vi "Max-Min2.vi"(0 "Color Plane (Color Plane Extraction 1)":i32(ring)=3 items=["Red", "Green", "Blue", "Hue", "Saturation", "Luminance", "Value", "Intensity"], 1 "Operator (Lookup Table 1)":T2(ring)=enum."Power X", 2 "X Value (Lookup Table 1)":sgl=2.0, 3 "ROI Descriptors (Quantify 1)":T1(array[cluster])=[{"Global Rectangle"=[0, 0, 160, 120], "Contours"=[{"ID"=enum."External", "Type"=3, "Coordinates"=[0, 0, 160, 120]}]}, {"Global Rectangle"=[18, 13, 28, 23], "Contours"=[{"ID"=enum."External", "Type"=3, "Coordinates"=[18, 13, 28, 23]}]}, {"Global Rectangle"=[77, 13, 87, 23], "Contours"=[{"ID"=enum."External", "Type"=3, "Coordinates"=[77, 13, 87, 23]}]}, {"Global Rectangle"=[135, 12, 145, 23], "Contours"=[{"ID"=enum."External", "Type"=3, "Coordinates"=[135, 12, 145, 23]}]}, {"Global Rectangle"=[18, 53, 28, 64], "Contours"=[{"ID"=enum."External", "Type"=3, "Coordinates"=[18, 53, 28, 64]}]}, {"Global Rectangle"=[77, 53, 87, 64], "Contours"=[{"ID"=enum."External", "Type"=3, "Coordinates"=[77, 53, 87, 64]}]}, {"Global Rectangle"=[137, 54, 146, 64], "Contours"=[{"ID"=enum."External", "Type"=3, "Coordinates"=[137, 54, 146, 64]}]}, {"Global Rectangle"=[18, 92, 28, 102], "Contours"=[{"ID"=enum."External", "Type"=3, "Coordinates"=[18, 92, 28, 102]}]}, {"Global Rectangle"=[77, 90, 87, 100], "Contours"=[{"ID"=enum."External", "Type"=3, "Coordinates"=[77, 90, 87, 100]}]}, {"Global Rectangle"=[136, 88, 146, 99], "Contours"=[{"ID"=enum."External", "Type"=3, "Coordinates"=[136, 88, 146, 99]}]}] {"Contours"."Type" items=["No Selection", "Point", "Line", "Rectangle", "Oval", "Polygon", "Freehand Region", "Annulus", "Unused2", "Unused3", "Broken Line", "Freehand Line", "Rotated Rectangle"]}, 7 "error in":errorcluster) -> (20 "Results (Quantify 1)":sgl[][](array[numeric]) format="%.2f", 27 "error out":errorcluster)   [LabVIEW 2009]
uses:
  <vilib>/vision/NI_Vision_Development_Module.lvlib
panel:
  out "Image Out":T3(plugin-control)
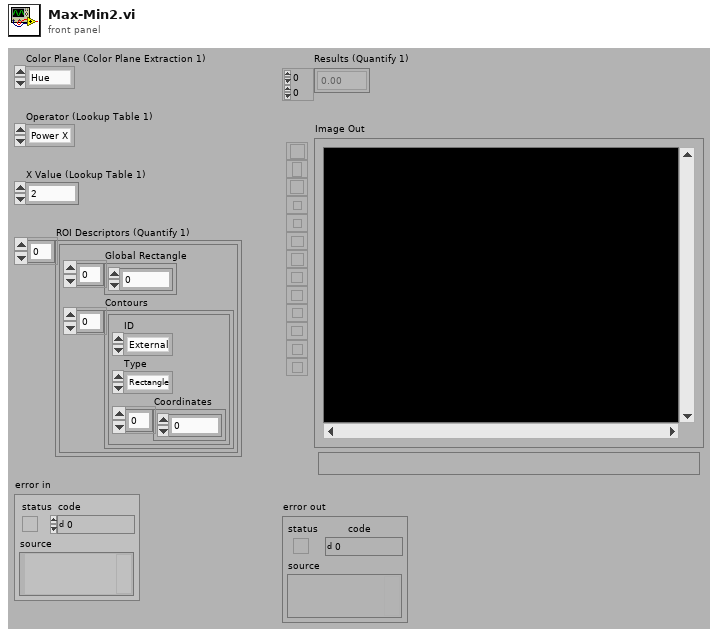
[diagram p1: front panel]
types:
  T1 = cluster{"Global Rectangle":i32[], "Contours":cluster{"ID":enum32{"External", "Internal"}, "Type":u32, "Coordinates":i32[]}[]}[]
  T2 = enum32{"Linear", "Log", "Exp", "Square", "Square root", "Power X", "Power 1/X"}
  T3 = typedef "IMAQ Image.ctl" = refnum<image>
  T4 = typedef "Image Type" = u32
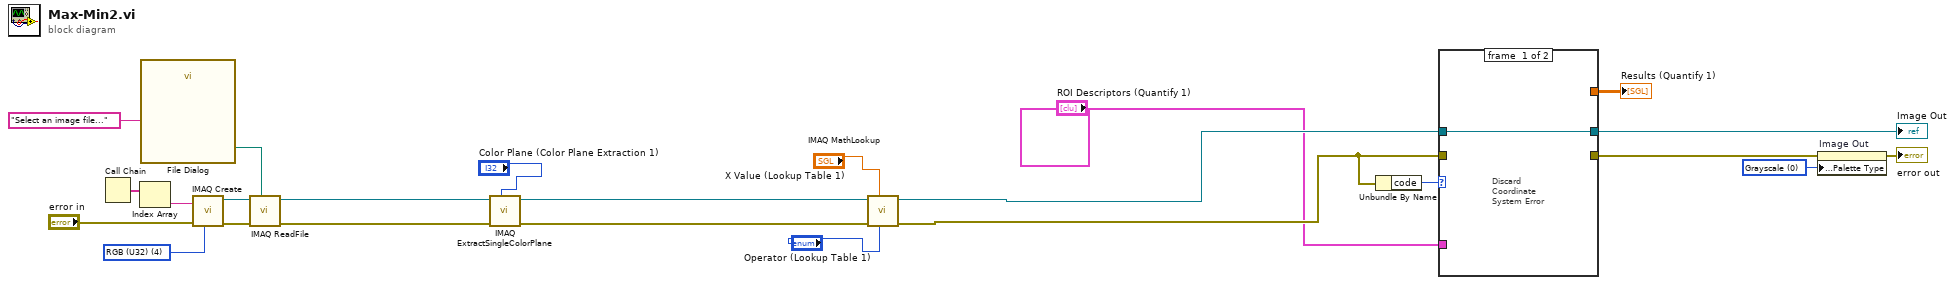
[diagram p0: block diagram]
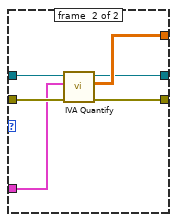
[diagram p2: hidden frame]
diagram:
  w2 = u32 0 items=["Grayscale", "Binary", "Gradient", "Rainbow", "Temperature", "User Defined"] ("Palette")
  w16 = T4 4 items=["Grayscale (U8)", "Grayscale (I16)", "Grayscale (SGL)", "Complex (CSG)", "RGB (U32)", "HSL (U32)", "RGB (U64)", "Grayscale (U16)"] ("Image Type")
  n1 = Call Chain() -> (call chain=w20:string[])
  n2 = Index Array(array=w20) -> (element=w19:string)  [unwired: 1 in]
  n3 = call "File Dialog"("prompt"="Select an image file...") -> ("selected path"=w17:path)  [unwired: 6 in, 8 out]
  n4 = call "IMAQ Create"("Image Name"=w19, "Image Type"=w16, "error in (no error)"="error in") -> ("New Image"=w23:T3, "error out"=w22:errorcluster)  [unwired: 1 in, 1 out]
  n5 = call "IMAQ ReadFile"("File Path"=w17, "error in (no error)"=w22, "Image"=w23) -> ("error out"=w24:errorcluster, "Image Out"=w14:T3)  [unwired: 2 in, 5 out]
  n6 = call "IMAQ ExtractSingleColorPlane"("Color Plane"="Color Plane (Color Plane Extraction 1)", "error in (no error)"=w24, "Image Src"=w14) -> ("error out"=w13:errorcluster, "Image Dst Out"=w10:T3)  [unwired: 1 in, 6 out]
  n7 = call "IMAQ MathLookup"("Operator"="Operator (Lookup Table 1)", "X Value"="X Value (Lookup Table 1)", "error in (no error)"=w13, "Image Src"=w10) -> ("error out"=w9:errorcluster, "Image Dst Out"=w7:T3)  [unwired: 3 in, 3 out]
  n8 = Unbundle By Name(w9) -> ("code"=w4:i32)
  n9 = case shown="Default" w4 {
    tunnel: [_ w31] -> w8
    tunnel: w7 -> [w25 w30]
    tunnel: w9 -> [_ w29]
    tunnel: [w25 w28] -> w3
    tunnel: [_ w27] -> w6
    tunnel: "ROI Descriptors (Quantify 1)" -> [_ w26]
    frame #0 {
      # "Discard\nCoordinate\nSystem Error"
    }
    frame #1 {
      n10 = call <vilib>:"IVA Quantify.vi"("error in (no error)"=w29, "ROI Descriptors"=w26, "Image"=w30) -> ("error out"=w27:errorcluster, "Results"=w31:sgl[][], "Image Out"=w28:T3)  [unwired: 6 out]
    }
  }
  "Results (Quantify 1)" <- w8
  "Image Out" <- w3
  n11 = property on="Image Out" class="ImageControl"(error in=w6, "Palette:Palette Type"=w2) -> (error out=→"error out":errorcluster)  [unwired: 1 in, 1 out]
